vi "GetClusterType.vi"(8 "error in":errorcluster, 11 "Control in":refnum<vi>) -> (0 "error out":errorcluster, 2 "Cluster Type":string, 3 "Control out":refnum<vi>)   [LabVIEW 2019]
doc: "9"
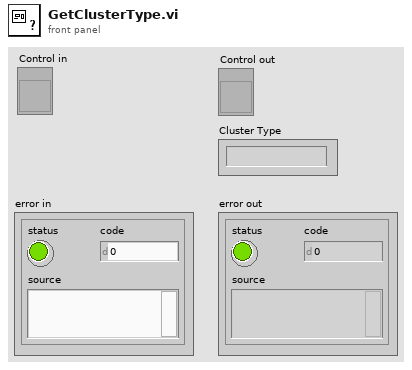
[diagram p1: front panel]
types:
  T1 = typedef "LVNumericRepresentation.ctl" = enum32{"Extended Precision", "Double Precision", "Single Precision", "Long", "Word", "Byte", "Unsigned Long", "Unsigned Word", "Unsigned Byte", "Complex Extended", "Complex Double", "Complex Single", "Quad", "Unsigned Quad", "Fixed-Point"}
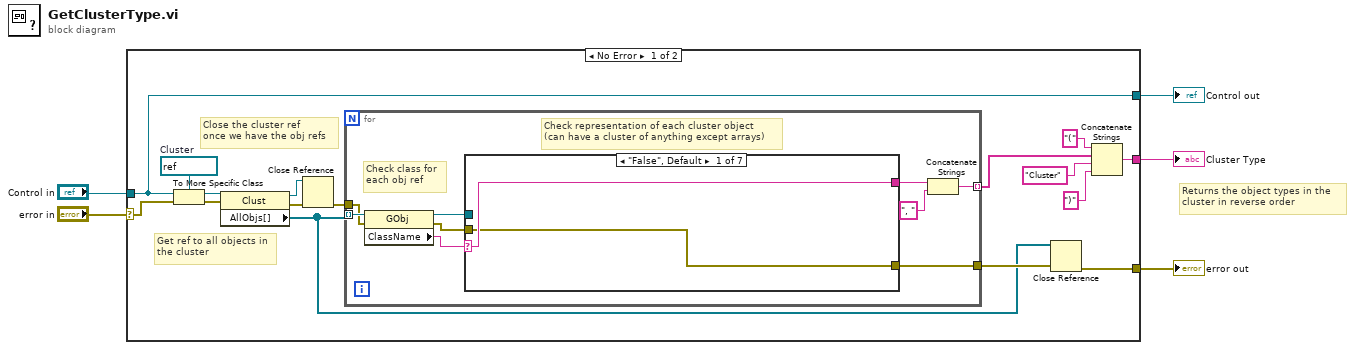
[diagram p0: block diagram]
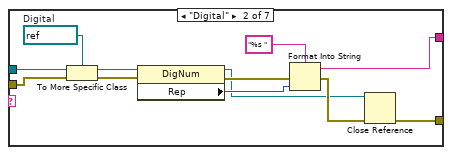
[diagram p2: hidden frame]
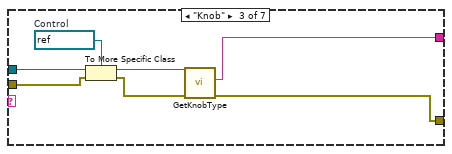
[diagram p3: hidden frame]
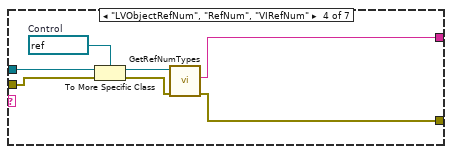
[diagram p4: hidden frame]
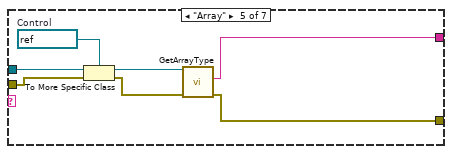
[diagram p5: hidden frame]
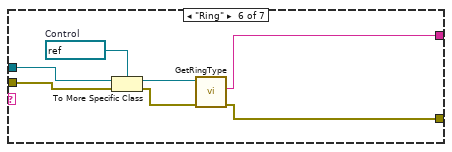
[diagram p6: hidden frame]
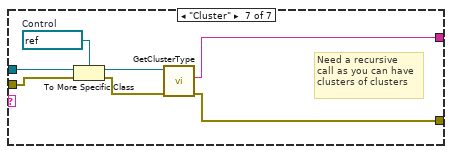
[diagram p7: hidden frame]
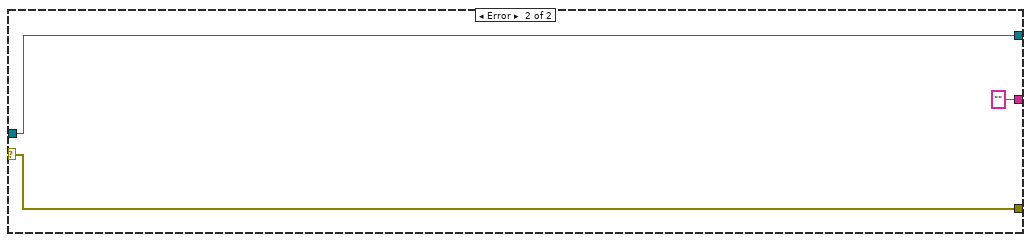
[diagram p8: hidden frame]
diagram:
  # "Returns the object types in the \ncluster in reverse order"
  n1 = case shown="No Error" "error in" {
    selector: "error in" -> [w12 w82]
    tunnel: "Control in" -> [w11 w80]
    tunnel: [w17 ""] -> w4
    tunnel: [w13 w82] -> w3
    tunnel: [w11 w80] -> w1
    frame No Error {
      w20 = refnum<vi> refnum  # Cluster
      # "Close the cluster ref\nonce we have the obj refs"
      # "Get ref to all objects in\nthe cluster"
      n2 = To More Specific Class(target class=w20, reference=w11, error in=w12) -> (specific class reference=w18:refnum<vi>, error out=w19:errorcluster)
      n3 = property class="Clust"(reference=w18, error in=w19) -> (reference out=w10:refnum<vi>, error out=w9:errorcluster, "AllObjs[]"=w14:refnum<vi>[])
      n4 = Close Reference(reference=w10, error in (no error)=w9) -> (error out=w8:errorcluster)
      n5 = for {
        tunnel: w14 -> [w28] mode=indexing
        tunnel: [w27] -> w21 mode=indexing
        tunnel: [w23] -> w15
        tunnel: w8 -> [w22]
        # "Check representation of each cluster object \n(can have a cluster of anything except arrays)"
        # "Check class for\neach obj ref"
        n6 = property class="GObj"(reference=w28, error in=w22) -> (reference out=w26:refnum<vi>, error out=w25:errorcluster, "ClassName"=w30:string)
        n7 = case shown="\"False\", Default" w30 {
          selector: w30 -> [w32 _ _ _ _ _ _]
          tunnel: [w32 w39 w46 w52 w61 w66 w75] -> w29
          tunnel: w26 -> [_ w38 w50 w57 w65 w70 w79]
          tunnel: w25 -> [w31 w37 w48 w56 w60 w71 w74]
          tunnel: [w31 w34 w45 w53 w62 w67 w76] -> w23
          frame "False", Default {
          }
          frame "Digital" {
            w42 = refnum<vi> refnum  # Digital
            n8 = To More Specific Class(target class=w42, reference=w38, error in=w37) -> (specific class reference=w44:refnum<vi>, error out=w43:errorcluster)
            n9 = property class="DigNum"(reference=w44, error in=w43) -> (reference out=w33:refnum<vi>, error out=w36:errorcluster, "Rep"=w40:T1)
            n10 = Format Into String(format string="%s ", error in=w36, w40) -> (resulting string=w39:string, error out=w35:errorcluster)  [unwired: 1 in]
            n11 = Close Reference(reference=w33, error in (no error)=w35) -> (error out=w34:errorcluster)
          }
          frame "Knob" {
            w51 = refnum<vi> refnum  # Control
            n12 = To More Specific Class(target class=w51, reference=w50, error in=w48) -> (specific class reference=w49:refnum<vi>, error out=w47:errorcluster)
            n13 = call "GetKnobType.vi"("error in (no error)"=w47, "reference in"=w49) -> ("error out"=w45:errorcluster, "Knob Type"=w46:string)  [unwired: 7 in, 1 out]
          }
          frame "LVObjectRefNum", "RefNum", "VIRefNum" {
            w58 = refnum<vi> refnum  # Control
            n14 = To More Specific Class(target class=w58, reference=w57, error in=w56) -> (specific class reference=w55:refnum<vi>, error out=w54:errorcluster)
            n15 = call "GetRefNumTypes.vi"("error in (no error)"=w54, "Control in"=w55) -> ("error out"=w53:errorcluster, "RefNumType"=w52:string)  [unwired: 7 in, 1 out]
          }
          frame "Array" {
            w63 = refnum<vi> refnum  # Control
            n16 = To More Specific Class(target class=w63, reference=w65, error in=w60) -> (specific class reference=w64:refnum<vi>, error out=w59:errorcluster)
            n17 = call "GetArrayType.vi"("error in (no error)"=w59, "Control in"=w64) -> ("error out"=w62:errorcluster, "Type"=w61:string)  [unwired: 7 in, 1 out]
          }
          frame "Ring" {
            w72 = refnum<vi> refnum  # Control
            n18 = To More Specific Class(target class=w72, reference=w70, error in=w71) -> (specific class reference=w69:refnum<vi>, error out=w68:errorcluster)
            n19 = call "GetRingType.vi"("error in (no error)"=w68, "Control Ref In"=w69) -> ("error out"=w67:errorcluster, "Ring Type"=w66:string)  [unwired: 7 in, 1 out]
          }
          frame "Cluster" {
            w77 = refnum<vi> refnum  # Control
            # "Need a recursive\ncall as you can have\nclusters of clusters"
            n20 = To More Specific Class(target class=w77, reference=w79, error in=w74) -> (specific class reference=w78:refnum<vi>, error out=w73:errorcluster)
            n21 = call "GetClusterType.vi"("error in"=w73, "Control in"=w78) -> ("error out"=w76:errorcluster, "Cluster Type"=w75:string)  [unwired: 7 in, 1 out]
          }
        }
        n22 = Concatenate Strings(w29, ", " ("string")) -> (w27:string)
      }
      n23 = Close Reference(reference=w14, error in (no error)=w15) -> (error out=w13:errorcluster)
      n24 = Concatenate Strings("(" ("string"), w21, "Cluster" ("string"), ")" ("string")) -> (w17:string)
    }
    frame Error {
    }
  }
  "Cluster Type" <- w4
  "error out" <- w3
  "Control out" <- w1
